vi "Version to Number.vi"(10 "error in":errorcluster, 11 "Web File Version in":string) -> (2 "error out":errorcluster, 3 "result":i32)   [LabVIEW 2013, in "main.lvlib"]
uses:
  main.lvlib
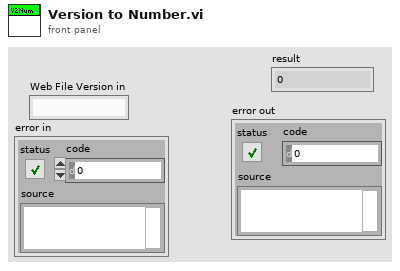
[diagram p1: front panel]
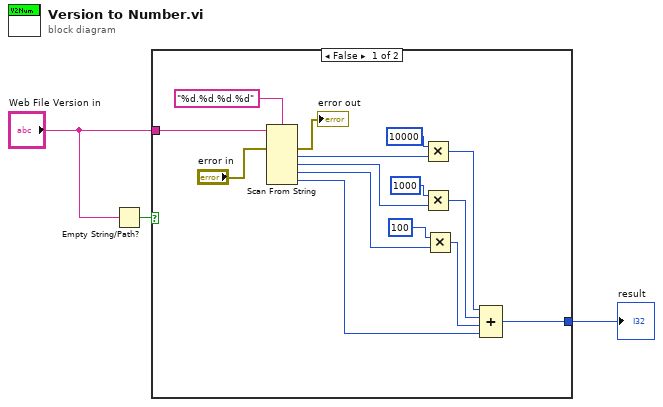
[diagram p0: block diagram]
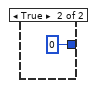
[diagram p2: hidden frame]
diagram:
  n1 = Empty String/Path?(string/path="Web File Version in") -> (empty?=w2:bool)
  n2 = case shown="False" w2 {
    tunnel: "Web File Version in" -> [w18 _]
    tunnel: [w16 0] -> w3
    frame False {
      n3 = Scan From String(format string="%d.%d.%d.%d", input string=w18, error in="error in") -> (error out=→"error out":errorcluster, output 1=w15:i32, output 2=w12:i32, output 3=w10:i32, output 4=w6:i32)  [unwired: 5 in, 2 out]
      n4 = Multiply(x=10000, y=w15) -> (x*y=w9:i32)
      n5 = Multiply(x=1000, y=w12) -> (x*y=w8:i32)
      n6 = Multiply(x=100, y=w10) -> (x*y=w7:i32)
      n7 = Compound Arithmetic op=ADD(w9, w8, w7, w6) -> (w16:i32)
    }
    frame True {
    }
  }
  "result" <- w3
